vi "chooseCase.vi"(9 "Robot":refnum<class "Robot.lvclass">, 10 "Game in":refnum<class "Game.lvclass">, 11 "Utilities in":refnum<class "Utilities.lvclass">) -> (3 "States":enum16{"PassObserver", "Halt", "Exit"}(ring))   [LabVIEW 2023, in "PassObserverTactic.lvclass"]
uses:
  PassObserverTactic.lvclass
  Robot_class/Robot.lvclass
  C:/Users/lucio/Desktop/roboime/SSL_AI/Object_class/Object.lvclass
  Game_class/Game.lvclass
  Utilities_class/Utilities.lvclass
  Team_class/OffensivePlay.ctl
  Game_class/Game.lvclass/Game.ctl
  Team_class/Team.lvclass/Team.ctl
  Robot_class/roles.ctl
  Object_class/Object.lvclass/Object.ctl
  Parameters_class/Parameters.lvclass/Parameters.ctl
  Robot_class/Robot.lvclass/Robot.ctl
  Object_class/Read x.vi
  Object_class/Read y.vi
  Game_class/Read OffensiveTeam.vi
  Game_class/Read BallRef.vi
  Game_class/Read Parameters.lvclass.vi
  Game_class/Read FieldRef.vi
  Parameters_class/Read AttakingOurselves.vi
  Team_class/Read OffensivePlay.vi
  Team_class/Read RobotRef.vi
  Robot_class/Read tactic.vi
  Robot_class/Read dest_orientation.vi
  Ball_class/Ball.lvclass
  Ally_class/Ally.lvclass
  C:/Users/lucio/Desktop/roboime/SSL_AI/Team_class/Team.lvclass
  Parameters_class/Parameters.lvclass
  Field_class/Field.lvclass
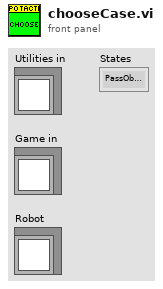
[diagram p1: front panel]
types:
  T1 = typedef "OffensivePlay.ctl" = enum16{"5RobotsPassGamePlay", "5PreparePassGame", "5RobotsKeeperGame", "KeeperPassToStriker", "5RobotsNormalGamePlay", "PrepareKeeperPass", "ACBPass", "ABCPass", "PrepareTriplePass", "TableWithStriker", "TableWith2ndStrikerPlay", "PrepareDoublePass", "PrepareRollToPass", "SimplePass", "PreparePass", "PassToStriker", "BallOutOfField", "PassTo2ndStriker", "StopOffensive", "Prepare Penalty Enemy", "EnemyPossessionAtEnemyField", "EnemyPossesionAtOurField", "TestPlay", "PreparePenaltyAlly", "KickPenaltyAlly", "PrepareKickoffAlly", "PrepareKickoffEnemy", "IndirectEnemy", "DirectEnemy", "PreparePassInGame1", "NormalGame", "DirectKick", "Pass", "Halt", "Timeout", "PassPlay", "PenaltyEnemy"}
  T2 = typedef "roles.ctl" = enum16{"SimpleBallPlacement", "BallPlacementAllyPasser", "BallPlacementAllyReceiver", "BallPlacementEnemy", "5Robots5th", "PassBestReceiver", "5Robots4th", "5Robots3rd", "5Robots2nd", "5Robots1st", "PassBestRobot", "WaitPass", "ABCThirdKicker", "ABCFirstKicker", "ABCSecondKicker", "Tabler", "TableFinalizer", "PrepareRollToPassRoller", "PrepareRollToPassReceiver", "SimplePassRoll", "SimplePassRollReceiver", "PenaltyDefense", "PreparePassReceiver 2", "PreparePassReceiver 1", "PassObserver", "Timeout", "Goto", "ZigZag", "None", "BallOutOfField", "DefenderArea", "Duelist", "AttackerStop", "FollowAttacker", "KeeperRole", "KickPenalty", "AttackerAimGoal", "AttackerBlock", "Marker", "Halt", "Shoot", "PassKicker", "PassReceiver", "TestRole", "PenaltyAttacker"}
  T3 = typedef "tactics.ctl" = enum16{"GoToBallPlacementPosition", "PlaceBall", "GoToBallPlacement", "5Robots", "BallPlacementEnemy", "ReceivePassInFuturePoint", "Roller", "PrepareRollToPassRollerGoTo", "PrepareRollToPassReceiverGoTo", "WaitRoll", "PositionToRoll", "PenaltyAttacker", "PassObserver", "PenaltyDefense", "TableReceiverTactic", "Test", "DefendGoal", "Marker", "FollowAttacker", "DefendArea", "Shoot", "AttackerAimGoal", "AttackerBallOutOfField", "AttackerBlock", "AttackerStop", "Duelist", "Halt", "ZigZag", "GoTo", "Timeout", "KickToBestRobot", "KickToPassReceiver", "PositionToReceivePass", "WaitPass", "GoToTarget"}
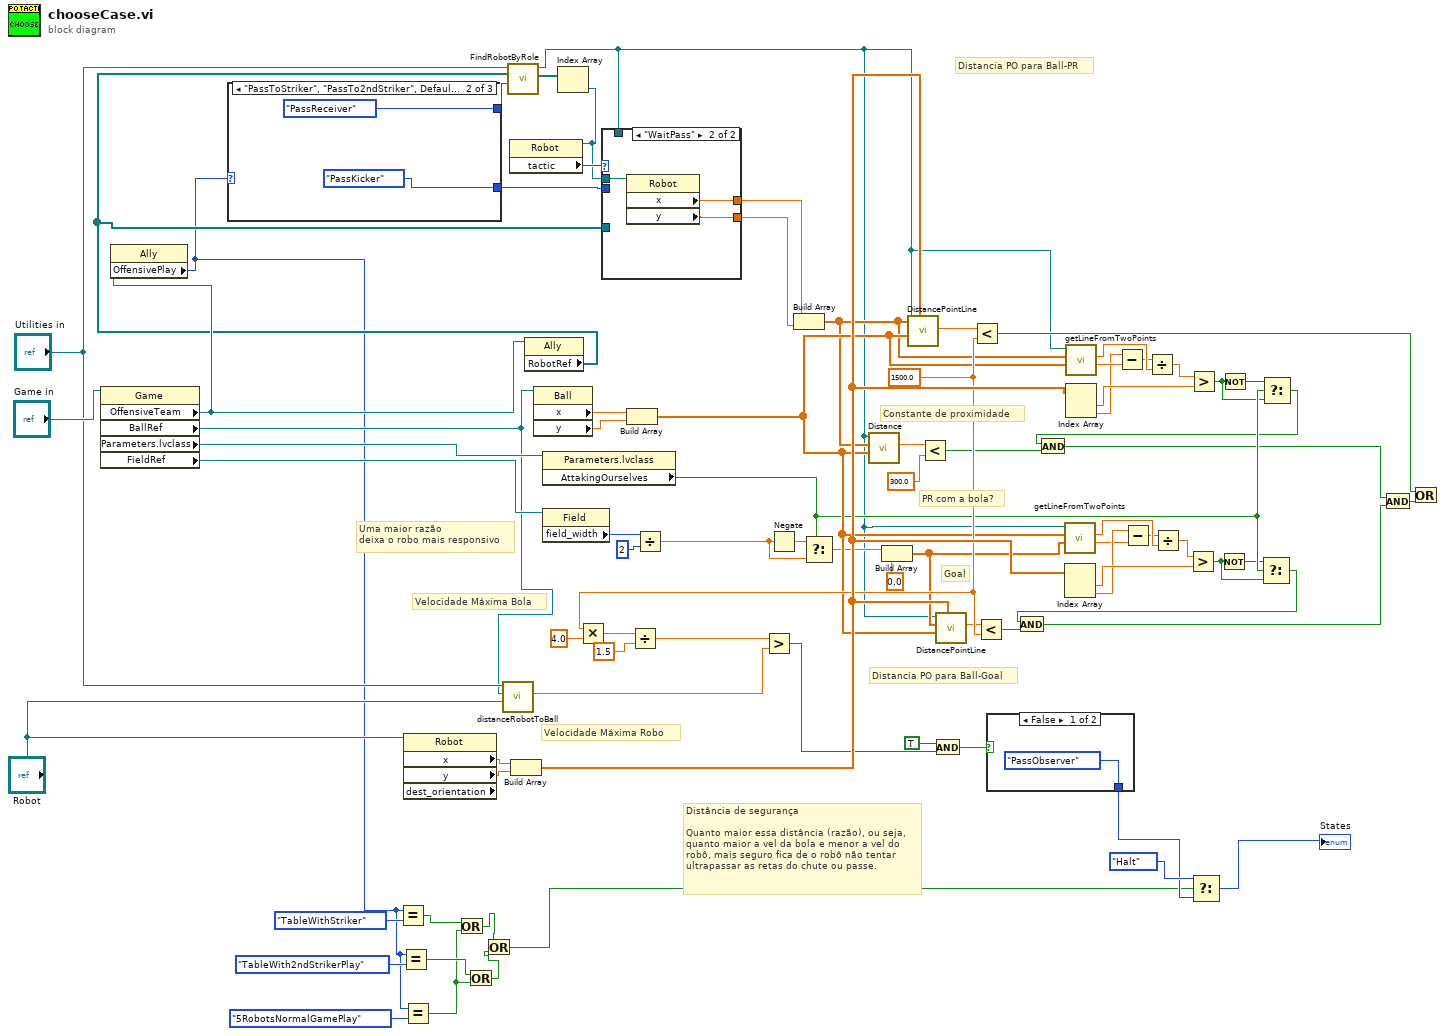
[diagram p0: block diagram]
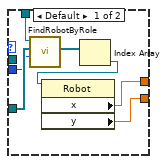
[diagram p2: hidden frame]
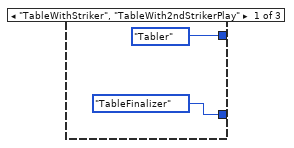
[diagram p3: hidden frame]
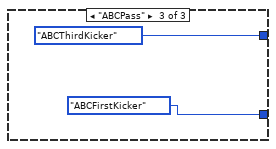
[diagram p4: hidden frame]
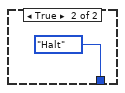
[diagram p5: hidden frame]
diagram:
  w68 = 1500.0 ("y")
  # "Uma maior razão\ndeixa o robo mais responsivo"
  # "PR com a bola?"
  # "Constante de proximidade"
  # "Distancia PO para Ball-Goal"
  # "Distancia PO para Ball-PR"
  # "Goal"
  # "Distância de segurança\n\nQuanto maior essa distância (razão), ou seja,\nquanto maior a vel da bola e menor a vel do\nrobô, mais seguro fica de o robô não tentar\nultrapassar as retas do chute ou passe."
  # "Velocidade Máxima Robo"
  # "Velocidade Máxima Bola"
  n1 = property class="Game"(reference="Game in") -> ("OffensiveTeam"=w22:refnum<class "Ally.lvclass">, "BallRef"=w23:refnum<class "Ball.lvclass">, "Parameters.lvclass"=w28:refnum<class "Parameters.lvclass">, "FieldRef"=w44:refnum<class "Field.lvclass">)  [unwired: 1 in, 2 out]
  n2 = property class="Ally"(reference=w22) -> ("OffensivePlay"=w7:T1)  [unwired: 1 in, 2 out]
  n3 = case shown="\"PassToStriker\", \"PassTo2ndStriker\", Default" w7 {
    tunnel: [roles."Tabler" ("role") roles."PassReceiver" ("role") roles."ABCThirdKicker" ("role")] -> w24
    tunnel: [roles."TableFinalizer" ("role") roles."PassKicker" ("role") roles."ABCFirstKicker" ("role")] -> w16
    frame "TableWithStriker", "TableWith2ndStrikerPlay" {
    }
    frame "PassToStriker", "PassTo2ndStriker", Default {
    }
    frame "ABCPass" {
    }
  }
  n4 = Equal?(x=w7, y=OffensivePlay."TableWithStriker") -> (x = y?=w11:bool)
  n5 = Equal?(x=w7, y=OffensivePlay."TableWith2ndStrikerPlay") -> (x = y?=w5:bool)
  n6 = Equal?(x=w7, y=OffensivePlay."5RobotsNormalGamePlay") -> (x = y?=w4:bool)
  n7 = property class="Robot" props=["x", "y", "dest_orientation"](reference="Robot") -> ("x"=w30:dbl, "y"=w26:dbl)  [unwired: 1 in, 3 out]
  n8 = Or(x=w11, y=w4) -> (x .or. y?=w2:bool)
  n9 = Or(x=w5, y=w4) -> (x .or. y?=w3:bool)
  n10 = Or(x=w2, y=w3) -> (x .or. y?=w1:bool)
  n11 = call "distanceRobotToBall.vi"("Robot"="Robot", "Ball"=w23, "Utilities in"="Utilities in") -> ("Distance Robot To Ball"=w40:dbl)  [unwired: 6 in, 2 out]
  n12 = Build Array(w30, w26) -> (w69:dbl[])
  n13 = property class="Ally"(reference=w22) -> ("RobotRef"=w17:refnum<class "Robot.lvclass">[])  [unwired: 1 in, 2 out]
  n14 = call "FindRobotByRole.vi"("role"=w24, "RobotRef"=w17, "Utilities in"="Utilities in") -> ("Robots"=w25:refnum<class "Robot.lvclass">[], "Utilities out"=w15:refnum<class "Utilities.lvclass">)  [unwired: 5 in, 2 out]
  n15 = property class="Ball"(reference=w23) -> ("x"=w31:dbl, "y"=w29:dbl)  [unwired: 1 in, 2 out]
  n16 = property class="Parameters.lvclass"(reference=w28) -> ("AttakingOurselves"=w64:bool)  [unwired: 1 in, 2 out]
  n17 = property class="Field"(reference=w44) -> ("field_width"=w45:i32)  [unwired: 1 in, 2 out]
  n18 = Index Array(array=w25) -> (element=w20:refnum<class "Robot.lvclass">)  [unwired: 1 in]
  n19 = property class="Robot"(reference=w20) -> ("tactic"=w21:T3)  [unwired: 1 in, 2 out]
  n20 = Multiply(x=w68, y=4.0) -> (x*y=w36:dbl)
  n21 = case shown="\"WaitPass\"" w21 {
    tunnel: w20 -> [_ w97]
    tunnel: [w89 w96] -> w19
    tunnel: [w88 w95] -> w18
    tunnel: w17 -> [w94 _]
    tunnel: w16 -> [w93 _]
    tunnel: w15 -> [w92 _]
    frame Default {
      n22 = call "FindRobotByRole.vi"("role"=w93, "RobotRef"=w94, "Utilities in"=w92) -> ("Robots"=w91:refnum<class "Robot.lvclass">[])  [unwired: 5 in, 3 out]
      n23 = Index Array(array=w91) -> (element=w90:refnum<class "Robot.lvclass">)  [unwired: 1 in]
      n24 = property class="Robot"(reference=w90) -> ("x"=w89:dbl, "y"=w88:dbl)  [unwired: 1 in, 2 out]
    }
    frame "WaitPass" {
      n25 = property class="Robot"(reference=w97) -> ("x"=w96:dbl, "y"=w95:dbl)  [unwired: 1 in, 2 out]
    }
  }
  n26 = Build Array(w31, w29) -> (w67:dbl[])
  n27 = Divide(x=w36, y=1.5) -> (x/y=w38:dbl)
  n28 = Divide(x=w45, y=2) -> (x/y=w48:dbl)
  n29 = Greater?(x=w38, y=w40) -> (0:w39:bool)
  n30 = Negate(x=w48) -> (-x=w47:dbl)
  n31 = Build Array(w19, w18) -> (w58:dbl[])
  n32 = Select(t=w47, s=w64, f=w48) -> (s? t:f=w49:dbl)
  n33 = call "Distance.vi"("P1"=w67, "P2"=w58, "Utilities in"=w15) -> ("Distance"=w42:dbl)  [unwired: 6 in, 2 out]
  n34 = Build Array(w49, 0.0 ("element")) -> (w66:dbl[])
  n35 = call "DistancePointLine.vi"("Q"=w69, "P2"=w67, "P1"=w58, "Utilities in"=w15) -> ("distance"=w27:dbl)  [unwired: 4 in, 3 out]
  n36 = Less?(x=w42, y=300.0) -> (x < y?=w57:bool)
  n37 = And(x=TRUE, y=w39) -> (x .and. y?=w41:bool)
  n38 = call "DistancePointLine.vi"("Q"=w69, "P2"=w67, "P1"=w66, "Utilities in"=w15) -> ("distance"=w51:dbl)  [unwired: 4 in, 3 out]
  n39 = Less?(x=w27, y=w68) -> (x < y?=w53:bool)
  n40 = Less?(x=w51, y=w68) -> (x < y?=w54:bool)
  n41 = case shown="False" w41 {
    tunnel: [enum16{"PassObserver", "Halt", "Exit"}."PassObserver" ("States") enum16{"PassObserver", "Halt", "Exit"}."Halt" ("States")] -> w9
    frame False {
    }
    frame True {
    }
  }
  n42 = call "getLineFromTwoPoints.vi"("Point 2"=w66, "Point 1"=w67, "Utilities in"=w15) -> ("linear coef"=w78:dbl, "angular coef"=w80:dbl)  [unwired: 4 in, 3 out]
  n43 = Index Array(array=w69) -> (element #1=w81:dbl, element #2=w79:dbl)  [unwired: 2 in]
  n44 = call "getLineFromTwoPoints.vi"("Point 2"=w67, "Point 1"=w58, "Utilities in"=w15) -> ("linear coef"=w71:dbl, "angular coef"=w73:dbl)  [unwired: 4 in, 3 out]
  n45 = Index Array(array=w69) -> (element #1=w75:dbl, element #2=w70:dbl)  [unwired: 2 in]
  n46 = Subtract(x=w70, y=w71) -> (x-y=w72:dbl)
  n47 = Subtract(x=w79, y=w78) -> (x-y=w76:dbl)
  n48 = Divide(x=w72, y=w73) -> (x/y=w74:dbl)
  n49 = Divide(x=w76, y=w80) -> (x/y=w77:dbl)
  n50 = Greater?(x=w77, y=w81) -> (0:w63:bool)
  n51 = Greater?(x=w74, y=w75) -> (0:w60:bool)
  n52 = Select(t=enum16{"PassObserver", "Halt", "Exit"}."Halt" ("States"), s=w1, f=w9) -> (s? t:f=→"States":enum16{"PassObserver", "Halt", "Exit"})
  n53 = Not(x=w63) -> (.not. x?=w62:bool)
  n54 = Not(x=w60) -> (.not. x?=w59:bool)
  n55 = Select(t=w62, s=w64, f=w63) -> (s? t:f=w65:bool)
  n56 = And(x=w65, y=w54) -> (x .and. y?=w56:bool)
  n57 = Select(t=w59, s=w64, f=w60) -> (s? t:f=w61:bool)
  n58 = And(x=w61, y=w57) -> (x .and. y?=w55:bool)
  n59 = And(x=w55, y=w56) -> (x .and. y?=w52:bool)
  n60 = Or(x=w53, y=w52) -> ()  [unwired: 1 out]
